vi "Stereo Vision - Grid Feature Extraction.vi"(8 "error in (no error)":errorcluster, 11 "Image in":T3) -> (0 "error out":errorcluster, 1 "Reference Points":T1, 3 "Image (dup)":T3)   [LabVIEW 2014]
doc: "Extracts the features from the input grid image."
uses:
  <vilib>/vision/Image Controls.llb/IMAQ Image.ctl
  <vilib>/vision/Calibration.llb/Calibration Reference Points.ctl
  <vilib>/vision/NI_Vision_Development_Module.lvlib
panel:
  # "Overview: Extracts the features from the input grid image."
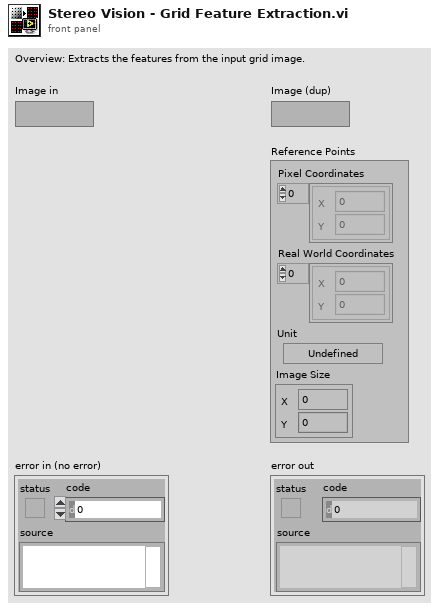
[diagram p1: front panel]
types:
  T1 = typedef "Calibration Reference Points.ctl" = cluster{"Pixel Coordinates":cluster{"X":dbl, "Y":dbl}[], "Real World Coordinates":cluster{"X":dbl, "Y":dbl}[], "Unit":T2, "Image Size":cluster{"X":u32, "Y":u32}}
  T2 = typedef "Image Unit" = enum32{"Undefined", "Angström", "Micrometer", "Millimeter", "Centimeter", "Meter", "Kilometer", "Microinch", "Inch", "Feet", "Nautical miles", "Standard miles", "Steps"}
  T3 = typedef "IMAQ Image.ctl" = refnum<image>
  T4 = typedef "Particle Parameters" = i32
  T5 = cluster{"Measurement Parameter":T4, "Range Lower Value":dbl, "Range Upper Value":dbl, "Range":bool, "Measurement Type":bool}[]
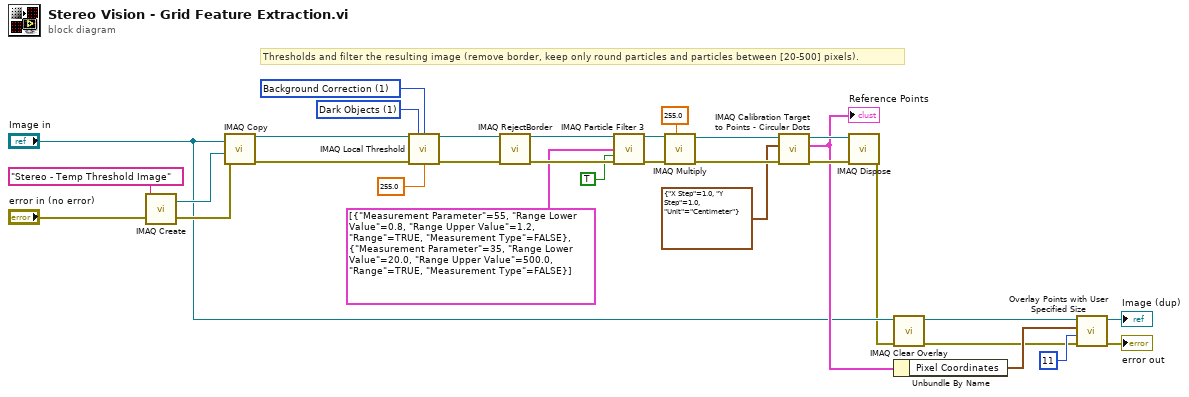
[diagram p0: block diagram]
diagram:
  w30 = u32 1 items=["Niblack", "Background Correction"] ("Method (Niblack)")
  w31 = u32 1 items=["Bright Objects", "Dark Objects"] ("Look For (Bright Objects)")
  # "Thresholds and filter the resulting image (remove border, keep only round particles and particles between [20-500] pixels)."
  n1 = call "IMAQ Create"("Image Name"="Stereo - Temp Threshold Image", "error in (no error)"="error in (no error)") -> ("New Image"=w23:T3, "error out"=w22:errorcluster)  [unwired: 2 in, 1 out]
  n2 = call "IMAQ Copy"("error in (no error)"=w22, "Image Dst"=w23, "Image Src"="Image in") -> ("error out"=w12:errorcluster, "Image Dst Out"=w15:T3)  [unwired: 3 out]
  n3 = call "IMAQ Local Threshold"("Image Src"=w15, "Look For (Bright Objects)"=w31, "Method (Niblack)"=w30, "error in (no error)"=w12, "Replace Value (1)"=sgl 255.0) -> ("Image Dst Out"=w28:T3, "error out"=w29:errorcluster)  [unwired: 3 in, 6 out]
  n4 = call "IMAQ RejectBorder"("error in (no error)"=w29, "Image Src"=w28) -> ("error out"=w26:errorcluster, "Image Dst Out"=w27:T3)  [unwired: 2 in, 2 out]
  n5 = call "IMAQ Particle Filter 3"("Image Src"=w27, "Selection Values"=T5 [{"Measurement Parameter"=55, "Range Lower Value"=0.8, "Range Upper Value"=1.2, "Range"=TRUE, "Measurement Type"=FALSE}, {"Measurement Parameter"=35, "Range Lower Value"=20.0, "Range Upper Value"=500.0, "Range"=TRUE, "Measurement Type"=FALSE}], "Keep/Remove Particles (F)"=TRUE, "error in (no error)"=w26) -> ("Image Dst Out"=w17:T3, "error out"=w19:errorcluster)  [unwired: 5 in, 5 out]
  n6 = call "IMAQ Multiply"("Image Src A"=w17, "Constant"=sgl 255.0, "error in (no error)"=w19) -> ("Image Dst Out"=w16:T3, "error out"=w18:errorcluster)  [unwired: 2 in, 2 out]
  n7 = call "IMAQ Calibration Target to Points - Circular Dots"("error in (no error)"=w18, "Grid Descriptor"=cluster{"X Step":sgl, "Y Step":sgl, "Unit":T2} {"X Step"=1.0, "Y Step"=1.0, "Unit"=enum."Centimeter"}, "Target Image"=w16) -> ("error out"=w10:errorcluster, "Reference Points"=w9:T1, "Target Image (dup)"=w21:T3)  [unwired: 2 in, 4 out]
  "Reference Points" <- w9
  n8 = call "IMAQ Dispose"("Image"=w21, "error in (no error)"=w10) -> ("error out"=w7:errorcluster)  [unwired: 1 in, 3 out]
  n9 = call "IMAQ Clear Overlay"("error in (no error)"=w7, "Image"="Image in") -> ("error out"=w2:errorcluster, "Image Out"=w3:T3)  [unwired: 1 in, 7 out]
  n10 = Unbundle By Name(w9) -> ("Pixel Coordinates"=w6:cluster{"X":dbl, "Y":dbl}[])
  n11 = call "Overlay Points with User Specified Size.vi"("error in"=w2, "Point Diameter (5)"=u32 11 ("Point Size (5)"), "Points"=w6, "Image In"=w3) -> ("error out"=→"error out":errorcluster, "Image Out"=→"Image (dup)":T3)  [unwired: 6 in]
